vi "Running Average.vi"(8 "error in (no error)":errorcluster caption="entrée d'erreur (pas d'erreur)") -> (0 "error out":errorcluster caption="sortie d'erreur")   [LabVIEW 2019, in "Calculations.lvclass"]
uses:
  Calculations Class/Calculations.lvclass
  C:/Programmes Labview/LabScanV1A/DevicesClass/BaseDevice/BaseDevice.lvclass
  Calculations Class/Calculations.lvclass/Calculations.ctl
  DevicesClass/BaseDevice/Accessor/GetClassEvent.vi
panel:
  out "Calculations Out.lvclass":refnum<class "Calculations.lvclass">
  in  "Calculations.lvclass":refnum<class "Calculations.lvclass">
  in  "Tab":enum32{"Description", "Parameters"}(tab)
  out "CalcDescription":string="Perform a running average on the selected data source. The function will average the last n data samples, where n is the \"Sample Count\" parameter provided"
  in  "MiseAJour":bool
  in  "SampleCount":i32=2 caption="Sample Count" min=1 step=1
  out "CalcPanelName":string="Running Average"
  in  "EditorProgQ":refnum<queue>
  in  "EditorProgQEvent":refnum<user-event>
  in  "Stop":bool
  out "Init Program":bool
  # "Running Average"
  # "this MUST be present and labeled \"Stop\""
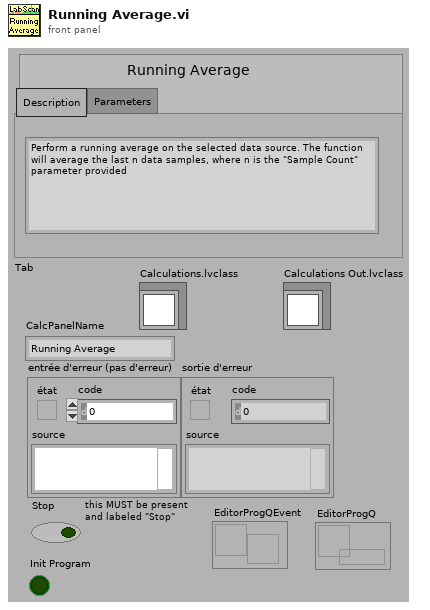
[diagram p1: front panel]
types:
  T1 = cluster{"Message":string, "Data":variant, "Code":i32}
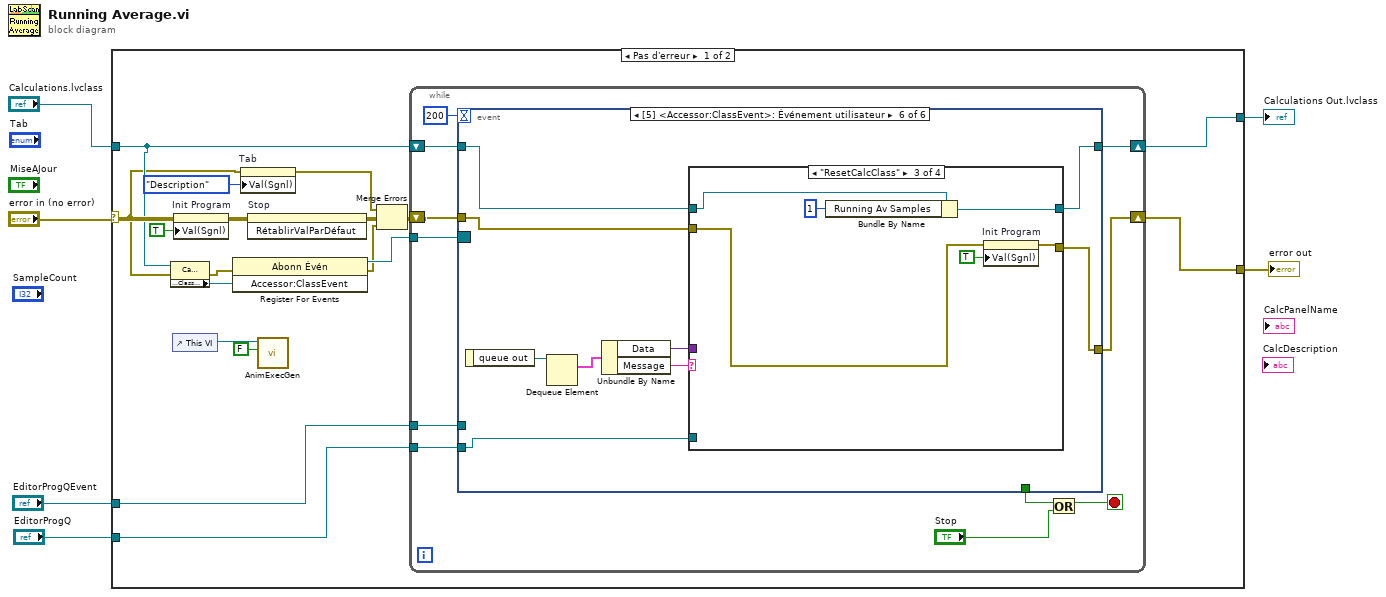
[diagram p0: block diagram]
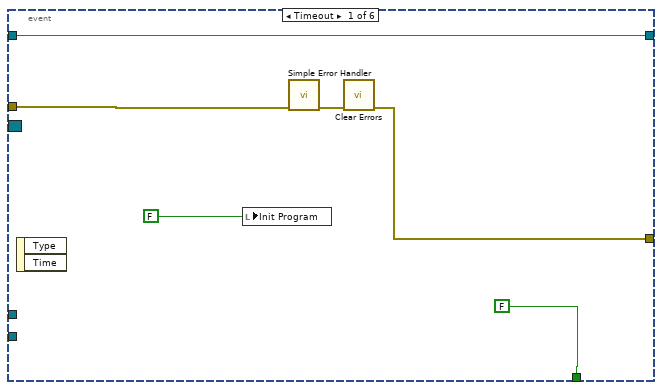
[diagram p2: hidden frame]
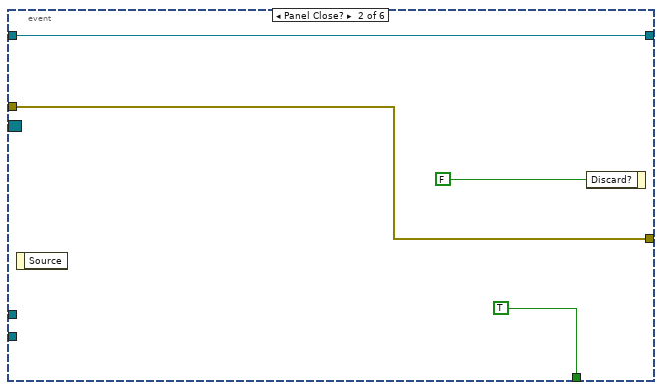
[diagram p3: hidden frame]
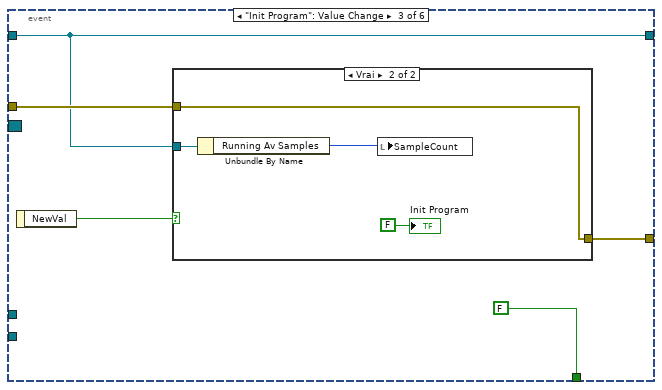
[diagram p4: hidden frame]
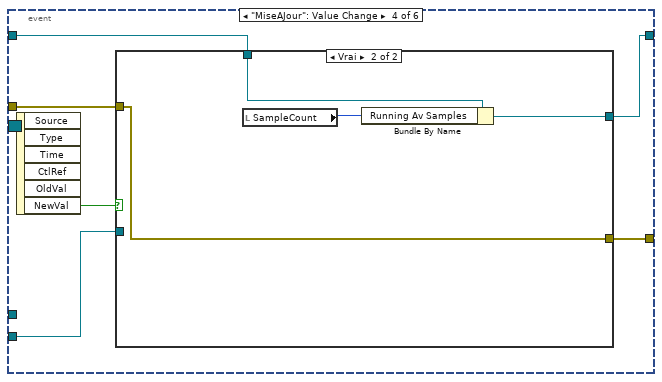
[diagram p6: hidden frame]
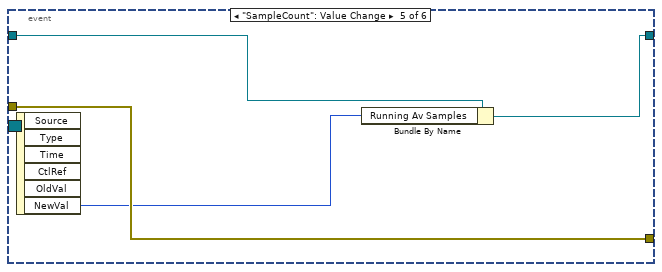
[diagram p8: hidden frame]
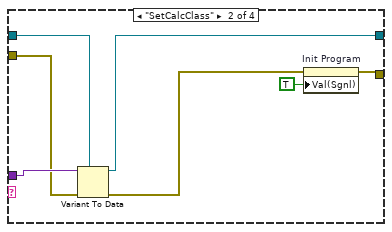
[diagram p10: hidden frame]
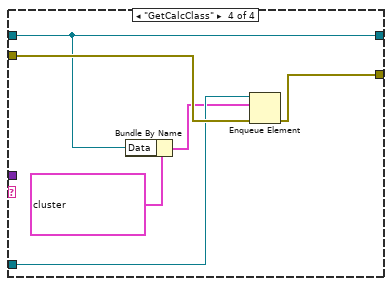
[diagram p11: hidden frame]
diagram:
  n1 = case shown="Pas d'erreur" "error in (no error)" {
    selector: "error in (no error)" -> [w10 w103]
    tunnel: [w24 w103] -> w5
    tunnel: "EditorProgQEvent" -> [w18 _]
    tunnel: "EditorProgQ" -> [w17 _]
    tunnel: "Calculations.lvclass" -> [w13 w102]
    tunnel: [w16 w102] -> w1
    frame No Error {
      n2 = property class="Calculations.lvclass"(reference=w13, error in=w10) -> (error out=w15:errorcluster, "Accessor:ClassEvent"=w14:refnum<user-event>)  [unwired: 1 out]
      n3 = control-ref of="This VI"() -> (w19:refnum<vi>)
      n4 = property on="Init Program" class="Bool (strict)"(error in=w10, "Val(Sgnl)"=TRUE ("Valeur (Signalisation)")) -> (error out=w22:errorcluster)  [unwired: 1 in, 1 out]
      n5 = register-events(error in=w15, w14) -> (reference out=w12:refnum<event-registration>, error out=w8:errorcluster)  [unwired: 1 in]
      n6 = property on="Tab" class="Onglet (strict)"(error in=w10, "Val(Sgnl)"=enum32{"Description", "Parameters"}."Description" ("Valeur (Signalisation)")) -> (error out=w7:errorcluster)  [unwired: 1 in, 1 out]
      n7 = invoke on="Stop" class="Bool (strict)" method="RétablirValParDéfaut"(error in=w22) -> (error out=w21:errorcluster)  [unwired: 2 in, 2 out]
      n8 = call <userlib>:"AnimExecGen.vi"("Animer l'exécution ?"=FALSE, "ViRef"=w19) -> ()  [unwired: 9 in, 1 out]
      n9 = Merge Errors(w7, w21, w8) -> (w9:errorcluster)
      n10 = while {
        shift-right: [w33] -> w24
        shift-left: w9 -> [w34]
        tunnel: w18 -> [w29]
        tunnel: w17 -> [w28]
        shift-right: [w26] -> w16
        shift-left: w13 -> [w27]
        tunnel: w12 -> [w25]
        stop <- w31 stop-if-true
        n11 = event shown="[5] <Accessor:ClassEvent>: Événement utilisateur" {
          selector: w25 -> [_ _ _ _ _ _]
          dyn-events: _ -> [_ _ _ _ _ _]
          timeout: 200 -> [_ _ _ _ _ _]
          tunnel: w34 -> [w40 w43 w49 w59 w70 w74]
          tunnel: [w38 w43 w48 w57 w70 w75] -> w33
          tunnel: [FALSE TRUE FALSE _ _ _] -> w32
          tunnel: w29 -> [_ _ _ _ _ _]
          tunnel: w28 -> [_ _ _ w60 _ w73]
          tunnel: w27 -> [w36 w42 w46 w58 w71 w77]
          tunnel: [w36 w42 w46 w56 w69 w76] -> w26
          event Timeout {
            n12 = event-data() -> ()  [unwired: 1 in, 2 out]
            n13 = local write "Init Program"(FALSE ("Init Program")) -> ()
            n14 = call <vilib>:"Simple Error Handler.vi"("error in (no error)"=w40) -> ("error out"=w39:errorcluster)  [unwired: 4 in, 4 out]
            n15 = call <vilib>:"Clear Errors.vi"("error in (no error)"=w39) -> ("error out"=w38:errorcluster)  [unwired: 5 in, 1 out]
          }
          event Panel Close? {
            n16 = event-data() -> ()  [unwired: 1 in, 1 out]
            n17 = event-data("Discard?"=FALSE ("Rejeter ?")) -> ()  [unwired: 1 in, 1 out]
          }
          event "Init Program": Value Change {
            n18 = event-data() -> ("NewVal"=w50:bool)  [unwired: 1 in]
            n19 = case shown="Vrai" w50 {
              tunnel: w49 -> [w51 w54]
              tunnel: [w51 w54] -> w48
              tunnel: w46 -> [_ w53]
              frame False {
              }
              frame True {
                n20 = Unbundle By Name(w53) -> ("Running Av Samples"=w52:i32)
                n21 = local write "SampleCount"(w52) -> ()
                "Init Program" <- FALSE
              }
            }
          }
          event "MiseAJour": Value Change {
            n22 = event-data() -> ("NewVal"=w61:bool)  [unwired: 1 in, 5 out]
            n23 = case shown="Vrai" w61 {
              tunnel: w58 -> [w62 w67]
              tunnel: w60 -> [_ _]
              tunnel: w59 -> [w63 w64]
              tunnel: [w63 w64] -> w57
              tunnel: [w62 w65] -> w56
              frame False {
              }
              frame True {
                n24 = local read "SampleCount"() -> (w66:i32)
                n25 = Bundle By Name(cluster=w67, "Running Av Samples"=w66) -> (w65:refnum<class "Calculations.lvclass">)
              }
            }
          }
          event "SampleCount": Value Change {
            n26 = event-data() -> ("NewVal"=w68:i32)  [unwired: 1 in, 5 out]
            n27 = Bundle By Name(cluster=w71, "Running Av Samples"=w68) -> (w69:refnum<class "Calculations.lvclass">)
          }
          event User Event {
            n28 = event-data() -> ("queue out"=w80:refnum<queue>)  [unwired: 1 in]
            n29 = Dequeue Element(queue=w80) -> (element=w79:cluster{"Message":string, "Data":variant, i32})  [unwired: 2 in, 3 out]
            n30 = Unbundle By Name(w79) -> ("Data"=w72:variant, "Message"=w78:string)
            n31 = case shown="\"ResetCalcClass\"" w78 {
              tunnel: w77 -> [w82 w86 w92 w96]
              tunnel: [w82 w85 w91 w96] -> w76
              tunnel: [w81 w88 w94 w97] -> w75
              tunnel: w74 -> [w81 w84 w93 w101]
              tunnel: w73 -> [_ _ _ w100]
              tunnel: w72 -> [_ w87 _ _]
              frame Default {
              }
              frame "SetCalcClass" {
                n32 = Variant To Data(error in=w84, type=w86, Variant=w87) -> (data=w85:refnum<class "Calculations.lvclass">, error out=w83:errorcluster)
                n33 = property on="Init Program" class="Bool (strict)"(error in=w83, "Val(Sgnl)"=TRUE ("Valeur (Signalisation)")) -> (error out=w88:errorcluster)  [unwired: 1 in, 1 out]
              }
              frame "ResetCalcClass" {
                n34 = Bundle By Name(cluster=w92, "Running Av Samples"=1) -> (w91:refnum<class "Calculations.lvclass">)
                n35 = property on="Init Program" class="Bool (strict)"(error in=w93, "Val(Sgnl)"=TRUE ("Valeur (Signalisation)")) -> (error out=w94:errorcluster)  [unwired: 1 in, 1 out]
              }
              frame "GetCalcClass" {
                n36 = Bundle By Name(cluster=T1 {"Message"="CalcClassExchange", "Data"=variant, "Code"=0} ("Message"), "Data"=w96) -> (w98:T1)
                n37 = Enqueue Element(queue=w100, element=w98, error in (no error)=w101) -> (error out=w97:errorcluster)  [unwired: 1 in, 2 out]
              }
            }
          }
        }
        n38 = Or(x=w32, y="Stop") -> (x .or. y?=w31:bool)
      }
    }
    frame Error {
    }
  }
  "error out" <- w5
  "Calculations Out.lvclass" <- w1
